vi "Set Pin Status.vi"(0 "Serial device in":refnum<class "Serial device.lvclass">, 5 "Port":dbl, 7 "Pin":dbl, 9 "Value":bool, 11 "error in (no error)":errorcluster) -> (4 "Serial device out":refnum<class "Serial device.lvclass">, 15 "error out":errorcluster)   [LabVIEW 2020, in "Serial device.lvclass"]
uses:
  Serial device.lvclass
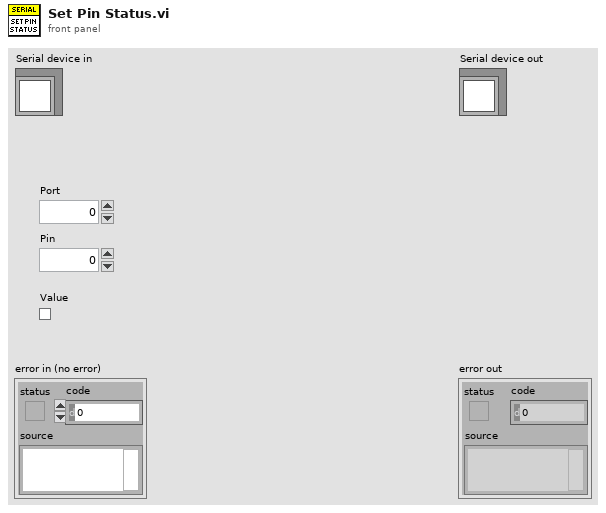
[diagram p1: front panel]
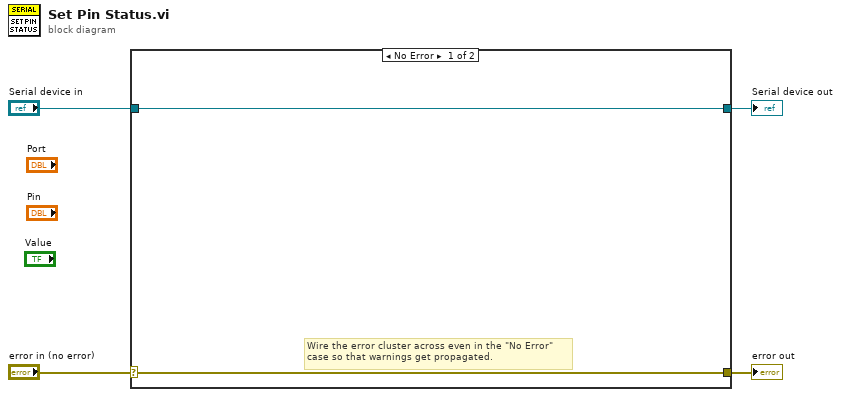
[diagram p0: block diagram]
diagram:
  n1 = case shown="No Error" "error in (no error)" {
    selector: "error in (no error)" -> [w5 w8]
    tunnel: [w5 w8] -> w3
    tunnel: [w6 w7] -> w1
    tunnel: "Serial device in" -> [w6 w7]
    frame No Error {
      # "Wire the error cluster across even in the \"No Error\"\ncase so that warnings get propagated."
    }
    frame Error {
    }
  }
  "error out" <- w3
  "Serial device out" <- w1
